vi "pp_trialTypes_codesUnique.vi"(11 "Trial Types":T1(array[cluster]) {"Stim P2" min=0.0; "Trial Weight" step=1; "Stim P1" min=0.0; "Stim Dur (s)" min=0.0; "Trial Code" min=1 step=1}) -> (0 "Code List":u16[](array[numeric]) min=1 step=1, 3 "Codes unique?":bool=TRUE)   [LabVIEW 2013]
uses:
  labolabo/array/impl/Unique_I.vi
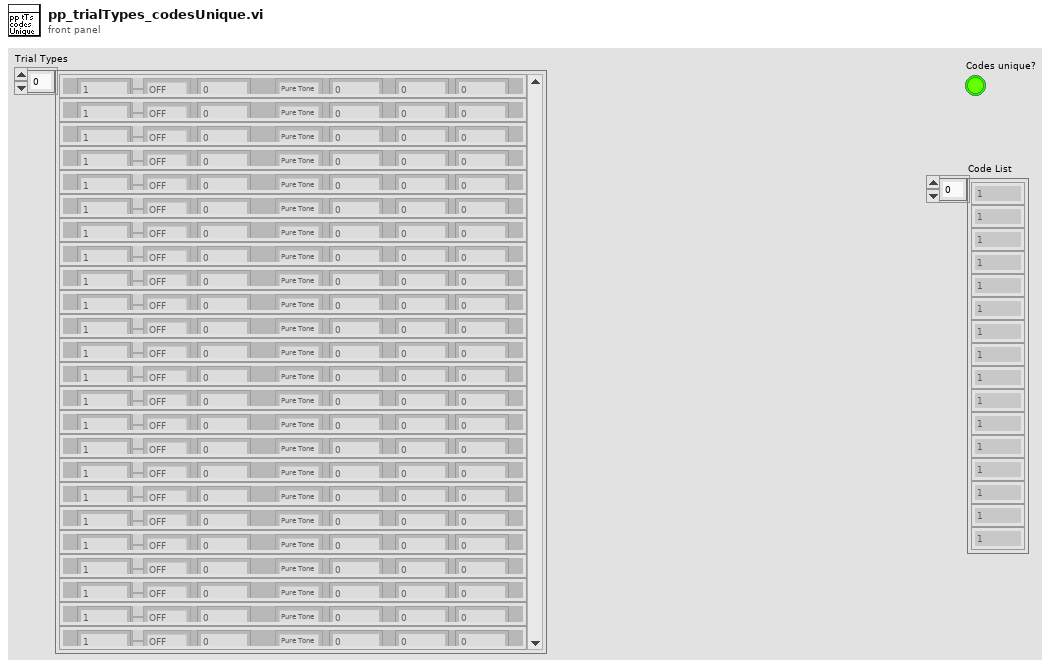
[diagram p1: front panel]
types:
  T1 = cluster{"Trial Code":u16, "Trial Type":enum16{"OFF", "GO", "NOGO", "TEST"}, "Trial Weight":u32, "Stim Type":enum16{"Pure Tone", "FM Sweep"}, "Stim Dur (s)":dbl, "Stim P1":dbl, "Stim P2":dbl}[]
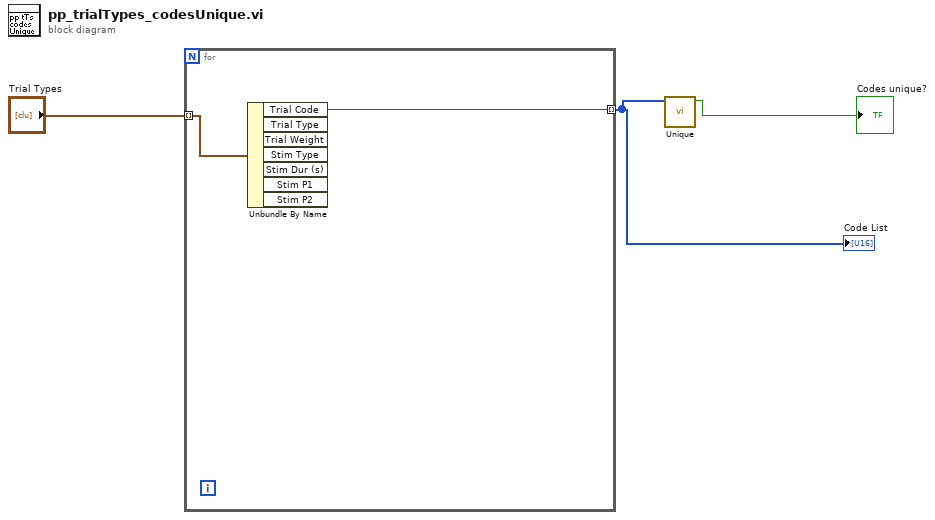
[diagram p0: block diagram]
diagram:
  n1 = for {
    tunnel: "Trial Types" -> [w5] mode=indexing
    tunnel: [w4] -> w1 mode=indexing
    n2 = Unbundle By Name(w5) -> ("Trial Code"=w4:u16)  [unwired: 6 out]
  }
  "Code List" <- w1
  n3 = call-poly "Unique.vi"("1D Array In"=w1) -> ("Boolean"=→"Codes unique?":bool)  [unwired: 10 in]
